vi "Lab Panel V5.11.vi"() -> ()   [LabVIEW 2013] (continued)
                      }
                    }
                    n1129 = Increment(x=w2164) -> (x+1=w2165:dbl)
                    n1130 = Greater Or Equal?(x=w2172, y=w2165) -> (x >= y?=w2174:bool)
                    n1131 = case shown="True" w2174 {
                      tunnel: w2169 -> [w2184 _]
                      tunnel: w2168 -> [w2183 _]
                      tunnel: w2167 -> [w2182 _]
                      tunnel: w2166 -> [w2181 _]
                      frame True {
                        n1132 = stacked-sequence {
                          tunnel: w2184 -> [w2188 _]
                          tunnel: w2183 -> [w2186 w2192]
                          tunnel: w2182 -> [_ w2195]
                          tunnel: w2181 -> [w2185 _]
                          frame #0 {
                            n1133 = Build Array(w2186) -> (w2189:string[])
                            n1134 = Build Array(w2188) -> (w2187:dbl[])
                            n1135 = TDMS Write(0:w2185, 5:"TEST PASS", 7:w2189, 9:w2187) -> (15:w2191:errorcluster)  [unwired: 2 in, 3 out]
                            n1136 = local write "data file error"(w2191) -> ()
                          }
                          frame #1 {
                            n1137 = Bundle(cluster=w2195, "STATUS"=w2192) -> (w2193:T4)  [unwired: 2 in]
                            n1138 = local write "RESULT LAB02-1"(TRUE) -> ()
                            n1139 = local write "DISP LAB02-1"(w2193) -> ()
                          }
                        }
                      }
                      frame False {
                      }
                    }
                  }
                }
              }
              frame #3 {
                # "LAB02-2"
                n1140 = Less?(x=w2196, y=2) -> (x < y?=w2199:bool)
                n1141 = local read "DISP LAB02-2"() -> (w2201:T4)
                n1142 = Unbundle(w2201) -> ("STATUS"=w2202:string)  [unwired: 2 out]
                n1143 = Equal?(x=w2202, y="RUN") -> (x = y?=w2198:bool)
                n1144 = And(x=w2198, y=w2199) -> (x .and. y?=w2197:bool)
                n1145 = case shown="True" w2197 {
                  tunnel: w2201 -> [_ w2207]
                  tunnel: w2196 -> [_ w2211]
                  frame False {
                  }
                  frame True {
                    n1146 = local read "SET LAB02-2"() -> (w2213:T5)
                    n1147 = local read "TDMS LAB02-2"() -> (w2206:refnum<k34>)
                    n1148 = Unbundle(w2207) -> ("CYCLE"=w2212:dbl)  [unwired: 2 out]
                    n1149 = Unbundle(w2213) -> ("CYCLES"=w2204:dbl, "T-RISE mins"=w2210:dbl)  [unwired: 3 out]
                    n1150 = case shown="\"T-RISE TEST\"" w2211 {
                      tunnel: w2210 -> [_ _ w2220]
                      tunnel: [w2215 w2217 w2220] -> w2209
                      tunnel: w2204 -> [w2215 w2217 _]
                      tunnel: ["CHART PASS" "CYCLE PASS" "T-RISE PASS"] -> w2208
                      frame "CHART TEST", Default {
                      }
                      frame "CYCLE TEST" {
                      }
                      frame "T-RISE TEST" {
                      }
                    }
                    n1151 = Increment(x=w2204) -> (x+1=w2205:dbl)
                    n1152 = Greater Or Equal?(x=w2212, y=w2205) -> (x >= y?=w2214:bool)
                    n1153 = case shown="True" w2214 {
                      tunnel: w2209 -> [w2224 _]
                      tunnel: w2208 -> [w2223 _]
                      tunnel: w2207 -> [w2222 _]
                      tunnel: w2206 -> [w2221 _]
                      frame True {
                        n1154 = stacked-sequence {
                          tunnel: w2224 -> [w2228 _]
                          tunnel: w2223 -> [w2226 w2232]
                          tunnel: w2222 -> [_ w2235]
                          tunnel: w2221 -> [w2225 _]
                          frame #0 {
                            n1155 = Build Array(w2226) -> (w2229:string[])
                            n1156 = Build Array(w2228) -> (w2227:dbl[])
                            n1157 = TDMS Write(0:w2225, 5:"TEST PASS", 7:w2229, 9:w2227) -> (15:w2231:errorcluster)  [unwired: 2 in, 3 out]
                            n1158 = local write "data file error"(w2231) -> ()
                          }
                          frame #1 {
                            n1159 = Bundle(cluster=w2235, "STATUS"=w2232) -> (w2233:T4)  [unwired: 2 in]
                            n1160 = local write "RESULT LAB02-2"(TRUE) -> ()
                            n1161 = local write "DISP LAB02-2"(w2233) -> ()
                          }
                        }
                      }
                      frame False {
                      }
                    }
                  }
                }
              }
              frame #4 {
                # "LAB03-1"
                n1162 = Less?(x=w2236, y=2) -> (x < y?=w2239:bool)
                n1163 = local read "DISP LAB03-1"() -> (w2241:T4)
                n1164 = Unbundle(w2241) -> ("STATUS"=w2242:string)  [unwired: 2 out]
                n1165 = Equal?(x=w2242, y="RUN") -> (x = y?=w2238:bool)
                n1166 = And(x=w2238, y=w2239) -> (x .and. y?=w2237:bool)
                n1167 = case shown="True" w2237 {
                  tunnel: w2241 -> [_ w2247]
                  tunnel: w2236 -> [_ w2251]
                  frame False {
                  }
                  frame True {
                    n1168 = local read "SET LAB03-1"() -> (w2253:T5)
                    n1169 = local read "TDMS LAB03-1"() -> (w2246:refnum<k34>)
                    n1170 = Unbundle(w2247) -> ("CYCLE"=w2252:dbl)  [unwired: 2 out]
                    n1171 = Unbundle(w2253) -> ("CYCLES"=w2244:dbl, "T-RISE mins"=w2250:dbl)  [unwired: 3 out]
                    n1172 = case shown="\"T-RISE TEST\"" w2251 {
                      tunnel: w2250 -> [_ _ w2260]
                      tunnel: [w2255 w2257 w2260] -> w2249
                      tunnel: w2244 -> [w2255 w2257 _]
                      tunnel: ["CHART PASS" "CYCLE PASS" "T-RISE PASS"] -> w2248
                      frame "CHART TEST", Default {
                      }
                      frame "CYCLE TEST" {
                      }
                      frame "T-RISE TEST" {
                      }
                    }
                    n1173 = Increment(x=w2244) -> (x+1=w2245:dbl)
                    n1174 = Greater Or Equal?(x=w2252, y=w2245) -> (x >= y?=w2254:bool)
                    n1175 = case shown="True" w2254 {
                      tunnel: w2249 -> [w2264 _]
                      tunnel: w2248 -> [w2263 _]
                      tunnel: w2247 -> [w2262 _]
                      tunnel: w2246 -> [w2261 _]
                      frame True {
                        n1176 = stacked-sequence {
                          tunnel: w2264 -> [w2268 _]
                          tunnel: w2263 -> [w2266 w2272]
                          tunnel: w2262 -> [_ w2275]
                          tunnel: w2261 -> [w2265 _]
                          frame #0 {
                            n1177 = Build Array(w2266) -> (w2269:string[])
                            n1178 = Build Array(w2268) -> (w2267:dbl[])
                            n1179 = TDMS Write(0:w2265, 5:"TEST PASS", 7:w2269, 9:w2267) -> (15:w2271:errorcluster)  [unwired: 2 in, 3 out]
                            n1180 = local write "data file error"(w2271) -> ()
                          }
                          frame #1 {
                            n1181 = Bundle(cluster=w2275, "STATUS"=w2272) -> (w2273:T4)  [unwired: 2 in]
                            n1182 = local write "RESULT LAB03-1"(TRUE) -> ()
                            n1183 = local write "DISP LAB03-1"(w2273) -> ()
                          }
                        }
                      }
                      frame False {
                      }
                    }
                  }
                }
              }
              frame #5 {
                # "LAB03-2"
                n1184 = Less?(x=w2276, y=2) -> (x < y?=w2279:bool)
                n1185 = local read "DISP LAB03-2"() -> (w2281:T4)
                n1186 = Unbundle(w2281) -> ("STATUS"=w2282:string)  [unwired: 2 out]
                n1187 = Equal?(x=w2282, y="RUN") -> (x = y?=w2278:bool)
                n1188 = And(x=w2278, y=w2279) -> (x .and. y?=w2277:bool)
                n1189 = case shown="True" w2277 {
                  tunnel: w2281 -> [_ w2287]
                  tunnel: w2276 -> [_ w2291]
                  frame False {
                  }
                  frame True {
                    n1190 = local read "SET LAB03-2"() -> (w2293:T5)
                    n1191 = local read "TDMS LAB03-2"() -> (w2286:refnum<k34>)
                    n1192 = Unbundle(w2287) -> ("CYCLE"=w2292:dbl)  [unwired: 2 out]
                    n1193 = Unbundle(w2293) -> ("CYCLES"=w2284:dbl, "T-RISE mins"=w2290:dbl)  [unwired: 3 out]
                    n1194 = case shown="\"T-RISE TEST\"" w2291 {
                      tunnel: w2290 -> [_ _ w2300]
                      tunnel: [w2295 w2297 w2300] -> w2289
                      tunnel: w2284 -> [w2295 w2297 _]
                      tunnel: ["CHART PASS" "CYCLE PASS" "T-RISE PASS"] -> w2288
                      frame "CHART TEST", Default {
                      }
                      frame "CYCLE TEST" {
                      }
                      frame "T-RISE TEST" {
                      }
                    }
                    n1195 = Increment(x=w2284) -> (x+1=w2285:dbl)
                    n1196 = Greater Or Equal?(x=w2292, y=w2285) -> (x >= y?=w2294:bool)
                    n1197 = case shown="True" w2294 {
                      tunnel: w2289 -> [w2304 _]
                      tunnel: w2288 -> [w2303 _]
                      tunnel: w2287 -> [w2302 _]
                      tunnel: w2286 -> [w2301 _]
                      frame True {
                        n1198 = stacked-sequence {
                          tunnel: w2304 -> [w2308 _]
                          tunnel: w2303 -> [w2306 w2312]
                          tunnel: w2302 -> [_ w2315]
                          tunnel: w2301 -> [w2305 _]
                          frame #0 {
                            n1199 = Build Array(w2306) -> (w2309:string[])
                            n1200 = Build Array(w2308) -> (w2307:dbl[])
                            n1201 = TDMS Write(0:w2305, 5:"TEST PASS", 7:w2309, 9:w2307) -> (15:w2311:errorcluster)  [unwired: 2 in, 3 out]
                            n1202 = local write "data file error"(w2311) -> ()
                          }
                          frame #1 {
                            n1203 = Bundle(cluster=w2315, "STATUS"=w2312) -> (w2313:T4)  [unwired: 2 in]
                            n1204 = local write "RESULT LAB03-2"(TRUE) -> ()
                            n1205 = local write "DISP LAB03-2"(w2313) -> ()
                          }
                        }
                      }
                      frame False {
                      }
                    }
                  }
                }
              }
              frame #6 {
                # "LAB04-1"
                n1206 = Less?(x=w2316, y=2) -> (x < y?=w2319:bool)
                n1207 = local read "DISP LAB04-1"() -> (w2321:T4)
                n1208 = Unbundle(w2321) -> ("STATUS"=w2322:string)  [unwired: 2 out]
                n1209 = Equal?(x=w2322, y="RUN") -> (x = y?=w2318:bool)
                n1210 = And(x=w2318, y=w2319) -> (x .and. y?=w2317:bool)
                n1211 = case shown="True" w2317 {
                  tunnel: w2321 -> [_ w2327]
                  tunnel: w2316 -> [_ w2331]
                  frame False {
                  }
                  frame True {
                    n1212 = local read "SET LAB04-1"() -> (w2333:T5)
                    n1213 = local read "TDMS LAB04-1"() -> (w2326:refnum<k34>)
                    n1214 = Unbundle(w2327) -> ("CYCLE"=w2332:dbl)  [unwired: 2 out]
                    n1215 = Unbundle(w2333) -> ("CYCLES"=w2324:dbl, "T-RISE mins"=w2330:dbl)  [unwired: 3 out]
                    n1216 = case shown="\"T-RISE TEST\"" w2331 {
                      tunnel: w2330 -> [_ _ w2340]
                      tunnel: [w2335 w2337 w2340] -> w2329
                      tunnel: w2324 -> [w2335 w2337 _]
                      tunnel: ["CHART PASS" "CYCLE PASS" "T-RISE PASS"] -> w2328
                      frame "CHART TEST", Default {
                      }
                      frame "CYCLE TEST" {
                      }
                      frame "T-RISE TEST" {
                      }
                    }
                    n1217 = Increment(x=w2324) -> (x+1=w2325:dbl)
                    n1218 = Greater Or Equal?(x=w2332, y=w2325) -> (x >= y?=w2334:bool)
                    n1219 = case shown="True" w2334 {
                      tunnel: w2329 -> [w2344 _]
                      tunnel: w2328 -> [w2343 _]
                      tunnel: w2327 -> [w2342 _]
                      tunnel: w2326 -> [w2341 _]
                      frame True {
                        n1220 = stacked-sequence {
                          tunnel: w2344 -> [w2348 _]
                          tunnel: w2343 -> [w2346 w2352]
                          tunnel: w2342 -> [_ w2355]
                          tunnel: w2341 -> [w2345 _]
                          frame #0 {
                            n1221 = Build Array(w2346) -> (w2349:string[])
                            n1222 = Build Array(w2348) -> (w2347:dbl[])
                            n1223 = TDMS Write(0:w2345, 5:"TEST PASS", 7:w2349, 9:w2347) -> (15:w2351:errorcluster)  [unwired: 2 in, 3 out]
                            n1224 = local write "data file error"(w2351) -> ()
                          }
                          frame #1 {
                            n1225 = Bundle(cluster=w2355, "STATUS"=w2352) -> (w2353:T4)  [unwired: 2 in]
                            n1226 = local write "RESULT LAB04-1"(TRUE) -> ()
                            n1227 = local write "DISP LAB04-1"(w2353) -> ()
                          }
                        }
                      }
                      frame False {
                      }
                    }
                  }
                }
              }
              frame #7 {
                # "LAB04-2"
                n1228 = Less?(x=w2356, y=2) -> (x < y?=w2359:bool)
                n1229 = local read "DISP LAB04-2"() -> (w2361:T4)
                n1230 = Unbundle(w2361) -> ("STATUS"=w2362:string)  [unwired: 2 out]
                n1231 = Equal?(x=w2362, y="RUN") -> (x = y?=w2358:bool)
                n1232 = And(x=w2358, y=w2359) -> (x .and. y?=w2357:bool)
                n1233 = case shown="True" w2357 {
                  tunnel: w2361 -> [_ w2367]
                  tunnel: w2356 -> [_ w2371]
                  frame False {
                  }
                  frame True {
                    n1234 = local read "SET LAB04-2"() -> (w2373:T5)
                    n1235 = local read "TDMS LAB04-2"() -> (w2366:refnum<k34>)
                    n1236 = Unbundle(w2367) -> ("CYCLE"=w2372:dbl)  [unwired: 2 out]
                    n1237 = Unbundle(w2373) -> ("CYCLES"=w2364:dbl, "T-RISE mins"=w2370:dbl)  [unwired: 3 out]
                    n1238 = case shown="\"T-RISE TEST\"" w2371 {
                      tunnel: w2370 -> [_ _ w2380]
                      tunnel: [w2375 w2377 w2380] -> w2369
                      tunnel: w2364 -> [w2375 w2377 _]
                      tunnel: ["CHART PASS" "CYCLE PASS" "T-RISE PASS"] -> w2368
                      frame "CHART TEST", Default {
                      }
                      frame "CYCLE TEST" {
                      }
                      frame "T-RISE TEST" {
                      }
                    }
                    n1239 = Increment(x=w2364) -> (x+1=w2365:dbl)
                    n1240 = Greater Or Equal?(x=w2372, y=w2365) -> (x >= y?=w2374:bool)
                    n1241 = case shown="True" w2374 {
                      tunnel: w2369 -> [w2384 _]
                      tunnel: w2368 -> [w2383 _]
                      tunnel: w2367 -> [w2382 _]
                      tunnel: w2366 -> [w2381 _]
                      frame True {
                        n1242 = stacked-sequence {
                          tunnel: w2384 -> [w2388 _]
                          tunnel: w2383 -> [w2386 w2392]
                          tunnel: w2382 -> [_ w2395]
                          tunnel: w2381 -> [w2385 _]
                          frame #0 {
                            n1243 = Build Array(w2386) -> (w2389:string[])
                            n1244 = Build Array(w2388) -> (w2387:dbl[])
                            n1245 = TDMS Write(0:w2385, 5:"TEST PASS", 7:w2389, 9:w2387) -> (15:w2391:errorcluster)  [unwired: 2 in, 3 out]
                            n1246 = local write "data file error"(w2391) -> ()
                          }
                          frame #1 {
                            n1247 = Bundle(cluster=w2395, "STATUS"=w2392) -> (w2393:T4)  [unwired: 2 in]
                            n1248 = local write "RESULT LAB04-2"(TRUE) -> ()
                            n1249 = local write "DISP LAB04-2"(w2393) -> ()
                          }
                        }
                      }
                      frame False {
                      }
                    }
                  }
                }
              }
              frame #8 {
                # "LAB05-1"
                n1250 = Less?(x=w2396, y=2) -> (x < y?=w2399:bool)
                n1251 = local read "DISP LAB05-1"() -> (w2401:T4)
                n1252 = Unbundle(w2401) -> ("STATUS"=w2402:string)  [unwired: 2 out]
                n1253 = Equal?(x=w2402, y="RUN") -> (x = y?=w2398:bool)
                n1254 = And(x=w2398, y=w2399) -> (x .and. y?=w2397:bool)
                n1255 = case shown="True" w2397 {
                  tunnel: w2401 -> [_ w2407]
                  tunnel: w2396 -> [_ w2411]
                  frame False {
                  }
                  frame True {
                    n1256 = local read "SET LAB05-1"() -> (w2413:T5)
                    n1257 = local read "TDMS LAB05-1"() -> (w2406:refnum<k34>)
                    n1258 = Unbundle(w2407) -> ("CYCLE"=w2412:dbl)  [unwired: 2 out]
                    n1259 = Unbundle(w2413) -> ("CYCLES"=w2404:dbl, "T-RISE mins"=w2410:dbl)  [unwired: 3 out]
                    n1260 = case shown="\"T-RISE TEST\"" w2411 {
                      tunnel: w2410 -> [_ _ w2420]
                      tunnel: [w2415 w2417 w2420] -> w2409
                      tunnel: w2404 -> [w2415 w2417 _]
                      tunnel: ["CHART PASS" "CYCLE PASS" "T-RISE PASS"] -> w2408
                      frame "CHART TEST", Default {
                      }
                      frame "CYCLE TEST" {
                      }
                      frame "T-RISE TEST" {
                      }
                    }
                    n1261 = Increment(x=w2404) -> (x+1=w2405:dbl)
                    n1262 = Greater Or Equal?(x=w2412, y=w2405) -> (x >= y?=w2414:bool)
                    n1263 = case shown="True" w2414 {
                      tunnel: w2409 -> [w2424 _]
                      tunnel: w2408 -> [w2423 _]
                      tunnel: w2407 -> [w2422 _]
                      tunnel: w2406 -> [w2421 _]
                      frame True {
                        n1264 = stacked-sequence {
                          tunnel: w2424 -> [w2428 _]
                          tunnel: w2423 -> [w2426 w2432]
                          tunnel: w2422 -> [_ w2435]
                          tunnel: w2421 -> [w2425 _]
                          frame #0 {
                            n1265 = Build Array(w2426) -> (w2429:string[])
                            n1266 = Build Array(w2428) -> (w2427:dbl[])
                            n1267 = TDMS Write(0:w2425, 5:"TEST PASS", 7:w2429, 9:w2427) -> (15:w2431:errorcluster)  [unwired: 2 in, 3 out]
                            n1268 = local write "data file error"(w2431) -> ()
                          }
                          frame #1 {
                            n1269 = Bundle(cluster=w2435, "STATUS"=w2432) -> (w2433:T4)  [unwired: 2 in]
                            n1270 = local write "RESULT LAB05-1"(TRUE) -> ()
                            n1271 = local write "DISP LAB05-1"(w2433) -> ()
                          }
                        }
                      }
                      frame False {
                      }
                    }
                  }
                }
              }
              frame #9 {
                # "LAB05-2"
                n1272 = Less?(x=w2436, y=2) -> (x < y?=w2439:bool)
                n1273 = local read "DISP LAB05-2"() -> (w2441:T4)
                n1274 = Unbundle(w2441) -> ("STATUS"=w2442:string)  [unwired: 2 out]
                n1275 = Equal?(x=w2442, y="RUN") -> (x = y?=w2438:bool)
                n1276 = And(x=w2438, y=w2439) -> (x .and. y?=w2437:bool)
                n1277 = case shown="True" w2437 {
                  tunnel: w2441 -> [_ w2447]
                  tunnel: w2436 -> [_ w2451]
                  frame False {
                  }
                  frame True {
                    n1278 = local read "SET LAB05-2"() -> (w2453:T5)
                    n1279 = local read "TDMS LAB05-2"() -> (w2446:refnum<k34>)
                    n1280 = Unbundle(w2447) -> ("CYCLE"=w2452:dbl)  [unwired: 2 out]
                    n1281 = Unbundle(w2453) -> ("CYCLES"=w2444:dbl, "T-RISE mins"=w2450:dbl)  [unwired: 3 out]
                    n1282 = case shown="\"T-RISE TEST\"" w2451 {
                      tunnel: w2450 -> [_ _ w2460]
                      tunnel: [w2455 w2457 w2460] -> w2449
                      tunnel: w2444 -> [w2455 w2457 _]
                      tunnel: ["CHART PASS" "CYCLE PASS" "T-RISE PASS"] -> w2448
                      frame "CHART TEST", Default {
                      }
                      frame "CYCLE TEST" {
                      }
                      frame "T-RISE TEST" {
                      }
                    }
                    n1283 = Increment(x=w2444) -> (x+1=w2445:dbl)
                    n1284 = Greater Or Equal?(x=w2452, y=w2445) -> (x >= y?=w2454:bool)
                    n1285 = case shown="True" w2454 {
                      tunnel: w2449 -> [w2464 _]
                      tunnel: w2448 -> [w2463 _]
                      tunnel: w2447 -> [w2462 _]
                      tunnel: w2446 -> [w2461 _]
                      frame True {
                        n1286 = stacked-sequence {
                          tunnel: w2464 -> [w2468 _]
                          tunnel: w2463 -> [w2466 w2472]
                          tunnel: w2462 -> [_ w2475]
                          tunnel: w2461 -> [w2465 _]
                          frame #0 {
                            n1287 = Build Array(w2466) -> (w2469:string[])
                            n1288 = Build Array(w2468) -> (w2467:dbl[])
                            n1289 = TDMS Write(0:w2465, 5:"TEST PASS", 7:w2469, 9:w2467) -> (15:w2471:errorcluster)  [unwired: 2 in, 3 out]
                            n1290 = local write "data file error"(w2471) -> ()
                          }
                          frame #1 {
                            n1291 = Bundle(cluster=w2475, "STATUS"=w2472) -> (w2473:T4)  [unwired: 2 in]
                            n1292 = local write "RESULT LAB05-2"(TRUE) -> ()
                            n1293 = local write "DISP LAB05-2"(w2473) -> ()
                          }
                        }
                      }
                      frame False {
                      }
                    }
                  }
                }
              }
            }
          }
          frame #5 {
            # "check if test cycles reached for temperature rise test"
            n1294 = stacked-sequence {
              tunnel: w2505 -> [_ _ _ _ _ _ _ _ _ _]
              tunnel: w2504 -> [_ _ _ _ _ _ _ _ _ _]
              tunnel: w2503 -> [_ _ _ _ _ _ _ _ _ _]
              tunnel: w2502 -> [_ _ _ _ _ _ _ _ _ _]
              tunnel: w2501 -> [_ _ _ _ _ _ _ _ _ _]
              tunnel: w2500 -> [_ _ _ _ _ _ _ _ _ _]
              tunnel: w2499 -> [_ _ _ _ _ _ _ _ _ _]
              tunnel: w2498 -> [_ _ _ _ _ _ _ _ _ _]
              tunnel: w2497 -> [_ _ _ _ _ _ _ _ _ _]
              tunnel: w2496 -> [_ _ _ _ _ _ _ _ _ _]
              tunnel: w2495 -> [w2511 _ _ _ _ _ _ _ _ _]
              tunnel: w2485 -> [w2506 _ _ _ _ _ _ _ _ _]
              tunnel: w2494 -> [_ w2537 _ _ _ _ _ _ _ _]
              tunnel: w2493 -> [_ _ w2567 _ _ _ _ _ _ _]
              tunnel: w2492 -> [_ _ _ w2597 _ _ _ _ _ _]
              tunnel: w2491 -> [_ _ _ _ w2627 _ _ _ _ _]
              tunnel: w2490 -> [_ _ _ _ _ w2657 _ _ _ _]
              tunnel: w2489 -> [_ _ _ _ _ _ w2687 _ _ _]
              tunnel: w2488 -> [_ _ _ _ _ _ _ w2717 _ _]
              tunnel: w2487 -> [_ _ _ _ _ _ _ _ w2747 _]
              tunnel: w2486 -> [_ _ _ _ _ _ _ _ _ w2777]
              tunnel: w2484 -> [_ w2536 _ _ _ _ _ _ _ _]
              tunnel: w2483 -> [_ _ w2566 _ _ _ _ _ _ _]
              tunnel: w2482 -> [_ _ _ w2596 _ _ _ _ _ _]
              tunnel: w2481 -> [_ _ _ _ w2626 _ _ _ _ _]
              tunnel: w2480 -> [_ _ _ _ _ w2656 _ _ _ _]
              tunnel: w2479 -> [_ _ _ _ _ _ w2686 _ _ _]
              tunnel: w2478 -> [_ _ _ _ _ _ _ w2716 _ _]
              tunnel: w2477 -> [_ _ _ _ _ _ _ _ w2746 _]
              tunnel: w2476 -> [_ _ _ _ _ _ _ _ _ w2776]
              frame #0 {
                # "LAB01-1"
                n1295 = Equal?(x=w2511, y=2) -> (x = y?=w2509:bool)
                n1296 = local read "DISP LAB01-1"() -> (w2512:T4)
                n1297 = Unbundle(w2512) -> ("STATUS"=w2513:string)  [unwired: 2 out]
                n1298 = Equal?(x=w2513, y="RUN") -> (x = y?=w2508:bool)
                n1299 = And(x=w2508, y=w2509) -> (x .and. y?=w2507:bool)
                n1300 = case shown="True" w2507 {
                  tunnel: w2512 -> [_ w2516]
                  tunnel: w2506 -> [_ w2519]
                  frame False {
                  }
                  frame True {
                    n1301 = local read "SET LAB01-1"() -> (w2518:T5)
                    n1302 = local read "TDMS LAB01-1"() -> (w2515:refnum<k34>)
                    n1303 = Unbundle(w2516) -> ("CYCLE"=w2520:dbl)  [unwired: 2 out]
                    n1304 = Unbundle(w2518) -> ("T-RISE mins"=w2517:dbl)  [unwired: 4 out]
                    n1305 = Greater Or Equal?(x=w2520, y=w2519) -> (x >= y?=w2521:bool)
                    n1306 = case shown="True" w2521 {
                      tunnel: w2517 -> [w2524 _]
                      tunnel: w2516 -> [w2523 _]
                      tunnel: w2515 -> [w2522 _]
                      frame True {
                        n1307 = stacked-sequence {
                          tunnel: w2524 -> [w2527 _]
                          tunnel: w2523 -> [_ w2532]
                          tunnel: w2522 -> [w2525 _]
                          frame #0 {
                            n1308 = Build Array("T-RISE") -> (w2529:string[])
                            n1309 = Build Array(w2527) -> (w2528:dbl[])
                            n1310 = TDMS Write(0:w2525, 5:"TEST PASS", 7:w2529, 9:w2528) -> (15:w2531:errorcluster)  [unwired: 2 in, 3 out]
                            n1311 = local write "data file error"(w2531) -> ()
                          }
                          frame #1 {
                            n1312 = Bundle(cluster=w2532, "STATUS"="T-RISE PASS") -> (w2534:T4)  [unwired: 2 in]
                            n1313 = local write "RESULT LAB01-1"(TRUE) -> ()
                            n1314 = local write "DISP LAB01-1"(w2534) -> ()
                          }
                        }
                      }
                      frame False {
                      }
                    }
                  }
                }
              }
              frame #1 {
                # "LAB01-2"
                n1315 = Equal?(x=w2537, y=2) -> (x = y?=w2540:bool)
                n1316 = local read "DISP LAB01-2"() -> (w2542:T4)
                n1317 = Unbundle(w2542) -> ("STATUS"=w2543:string)  [unwired: 2 out]
                n1318 = Equal?(x=w2543, y="RUN") -> (x = y?=w2539:bool)
                n1319 = And(x=w2539, y=w2540) -> (x .and. y?=w2538:bool)
                n1320 = case shown="True" w2538 {
                  tunnel: w2542 -> [_ w2546]
                  tunnel: w2536 -> [_ w2549]
                  frame False {
                  }
                  frame True {
                    n1321 = local read "SET LAB01-2"() -> (w2548:T5)
                    n1322 = local read "TDMS LAB01-2"() -> (w2545:refnum<k34>)
                    n1323 = Unbundle(w2546) -> ("CYCLE"=w2550:dbl)  [unwired: 2 out]
                    n1324 = Unbundle(w2548) -> ("T-RISE mins"=w2547:dbl)  [unwired: 4 out]
                    n1325 = Greater Or Equal?(x=w2550, y=w2549) -> (x >= y?=w2551:bool)
                    n1326 = case shown="True" w2551 {
                      tunnel: w2547 -> [w2554 _]
                      tunnel: w2546 -> [w2553 _]
                      tunnel: w2545 -> [w2552 _]
                      frame True {
                        n1327 = stacked-sequence {
                          tunnel: w2554 -> [w2557 _]
                          tunnel: w2553 -> [_ w2562]
                          tunnel: w2552 -> [w2555 _]
                          frame #0 {
                            n1328 = Build Array("T-RISE") -> (w2559:string[])
                            n1329 = Build Array(w2557) -> (w2558:dbl[])
                            n1330 = TDMS Write(0:w2555, 5:"TEST PASS", 7:w2559, 9:w2558) -> (15:w2561:errorcluster)  [unwired: 2 in, 3 out]
                            n1331 = local write "data file error"(w2561) -> ()
                          }
                          frame #1 {
                            n1332 = Bundle(cluster=w2562, "STATUS"="T-RISE PASS") -> (w2564:T4)  [unwired: 2 in]
                            n1333 = local write "RESULT LAB01-2"(TRUE) -> ()
                            n1334 = local write "DISP LAB01-2"(w2564) -> ()
                          }
                        }
                      }
                      frame False {
                      }
                    }
                  }
                }
              }
              frame #2 {
                # "LAB02-1"
                n1335 = Equal?(x=w2567, y=2) -> (x = y?=w2570:bool)
                n1336 = local read "DISP LAB02-1"() -> (w2572:T4)
                n1337 = Unbundle(w2572) -> ("STATUS"=w2573:string)  [unwired: 2 out]
                n1338 = Equal?(x=w2573, y="RUN") -> (x = y?=w2569:bool)
                n1339 = And(x=w2569, y=w2570) -> (x .and. y?=w2568:bool)
                n1340 = case shown="True" w2568 {
                  tunnel: w2572 -> [_ w2576]
                  tunnel: w2566 -> [_ w2579]
                  frame False {
                  }
                  frame True {
                    n1341 = local read "SET LAB02-1"() -> (w2578:T5)
                    n1342 = local read "TDMS LAB02-1"() -> (w2575:refnum<k34>)
                    n1343 = Unbundle(w2576) -> ("CYCLE"=w2580:dbl)  [unwired: 2 out]
                    n1344 = Unbundle(w2578) -> ("T-RISE mins"=w2577:dbl)  [unwired: 4 out]
                    n1345 = Greater Or Equal?(x=w2580, y=w2579) -> (x >= y?=w2581:bool)
                    n1346 = case shown="True" w2581 {
                      tunnel: w2577 -> [w2584 _]
                      tunnel: w2576 -> [w2583 _]
                      tunnel: w2575 -> [w2582 _]
                      frame True {
                        n1347 = stacked-sequence {
                          tunnel: w2584 -> [w2587 _]
                          tunnel: w2583 -> [_ w2592]
                          tunnel: w2582 -> [w2585 _]
                          frame #0 {
                            n1348 = Build Array("T-RISE") -> (w2589:string[])
                            n1349 = Build Array(w2587) -> (w2588:dbl[])
                            n1350 = TDMS Write(0:w2585, 5:"TEST PASS", 7:w2589, 9:w2588) -> (15:w2591:errorcluster)  [unwired: 2 in, 3 out]
                            n1351 = local write "data file error"(w2591) -> ()
                          }
                          frame #1 {
                            n1352 = Bundle(cluster=w2592, "STATUS"="T-RISE PASS") -> (w2594:T4)  [unwired: 2 in]
                            n1353 = local write "RESULT LAB02-1"(TRUE) -> ()
                            n1354 = local write "DISP LAB02-1"(w2594) -> ()
                          }
                        }
                      }
                      frame False {
                      }
                    }
                  }
                }
              }
              frame #3 {
                # "LAB02-2"
                n1355 = Equal?(x=w2597, y=2) -> (x = y?=w2600:bool)
                n1356 = local read "DISP LAB02-2"() -> (w2602:T4)
                n1357 = Unbundle(w2602) -> ("STATUS"=w2603:string)  [unwired: 2 out]
                n1358 = Equal?(x=w2603, y="RUN") -> (x = y?=w2599:bool)
                n1359 = And(x=w2599, y=w2600) -> (x .and. y?=w2598:bool)
                n1360 = case shown="True" w2598 {
                  tunnel: w2602 -> [_ w2606]
                  tunnel: w2596 -> [_ w2609]
                  frame False {
                  }
                  frame True {
                    n1361 = local read "SET LAB02-2"() -> (w2608:T5)
                    n1362 = local read "TDMS LAB02-2"() -> (w2605:refnum<k34>)
                    n1363 = Unbundle(w2606) -> ("CYCLE"=w2610:dbl)  [unwired: 2 out]
                    n1364 = Unbundle(w2608) -> ("T-RISE mins"=w2607:dbl)  [unwired: 4 out]
                    n1365 = Greater Or Equal?(x=w2610, y=w2609) -> (x >= y?=w2611:bool)
                    n1366 = case shown="True" w2611 {
                      tunnel: w2607 -> [w2614 _]
                      tunnel: w2606 -> [w2613 _]
                      tunnel: w2605 -> [w2612 _]
                      frame True {
                        n1367 = stacked-sequence {
                          tunnel: w2614 -> [w2617 _]
                          tunnel: w2613 -> [_ w2622]
                          tunnel: w2612 -> [w2615 _]
                          frame #0 {
                            n1368 = Build Array("T-RISE") -> (w2619:string[])
                            n1369 = Build Array(w2617) -> (w2618:dbl[])
                            n1370 = TDMS Write(0:w2615, 5:"TEST PASS", 7:w2619, 9:w2618) -> (15:w2621:errorcluster)  [unwired: 2 in, 3 out]
                            n1371 = local write "data file error"(w2621) -> ()
                          }
                          frame #1 {
                            n1372 = Bundle(cluster=w2622, "STATUS"="T-RISE PASS") -> (w2624:T4)  [unwired: 2 in]
                            n1373 = local write "RESULT LAB02-2"(TRUE) -> ()
                            n1374 = local write "DISP LAB02-2"(w2624) -> ()
                          }
                        }
                      }
                      frame False {
                      }
                    }
                  }
                }
              }
              frame #4 {
                # "LAB03-1"
                n1375 = Equal?(x=w2627, y=2) -> (x = y?=w2630:bool)
                n1376 = local read "DISP LAB03-1"() -> (w2632:T4)
                n1377 = Unbundle(w2632) -> ("STATUS"=w2633:string)  [unwired: 2 out]
                n1378 = Equal?(x=w2633, y="RUN") -> (x = y?=w2629:bool)
                n1379 = And(x=w2629, y=w2630) -> (x .and. y?=w2628:bool)
                n1380 = case shown="True" w2628 {
                  tunnel: w2632 -> [_ w2636]
                  tunnel: w2626 -> [_ w2639]
                  frame False {
                  }
                  frame True {
                    n1381 = local read "SET LAB03-1"() -> (w2638:T5)
                    n1382 = local read "TDMS LAB03-1"() -> (w2635:refnum<k34>)
                    n1383 = Unbundle(w2636) -> ("CYCLE"=w2640:dbl)  [unwired: 2 out]
                    n1384 = Unbundle(w2638) -> ("T-RISE mins"=w2637:dbl)  [unwired: 4 out]
                    n1385 = Greater Or Equal?(x=w2640, y=w2639) -> (x >= y?=w2641:bool)
                    n1386 = case shown="True" w2641 {
                      tunnel: w2637 -> [w2644 _]
                      tunnel: w2636 -> [w2643 _]
                      tunnel: w2635 -> [w2642 _]
                      frame True {
                        n1387 = stacked-sequence {
                          tunnel: w2644 -> [w2647 _]
                          tunnel: w2643 -> [_ w2652]
                          tunnel: w2642 -> [w2645 _]
                          frame #0 {
                            n1388 = Build Array("T-RISE") -> (w2649:string[])
                            n1389 = Build Array(w2647) -> (w2648:dbl[])
                            n1390 = TDMS Write(0:w2645, 5:"TEST PASS", 7:w2649, 9:w2648) -> (15:w2651:errorcluster)  [unwired: 2 in, 3 out]
                            n1391 = local write "data file error"(w2651) -> ()
                          }
                          frame #1 {
                            n1392 = Bundle(cluster=w2652, "STATUS"="T-RISE PASS") -> (w2654:T4)  [unwired: 2 in]
                            n1393 = local write "RESULT LAB03-1"(TRUE) -> ()
                            n1394 = local write "DISP LAB03-1"(w2654) -> ()
                          }
                        }
                      }
                      frame False {
                      }
                    }
                  }
                }
              }
              frame #5 {
                # "LAB03-2"
                n1395 = Equal?(x=w2657, y=2) -> (x = y?=w2660:bool)
                n1396 = local read "DISP LAB03-2"() -> (w2662:T4)
                n1397 = Unbundle(w2662) -> ("STATUS"=w2663:string)  [unwired: 2 out]
                n1398 = Equal?(x=w2663, y="RUN") -> (x = y?=w2659:bool)
                n1399 = And(x=w2659, y=w2660) -> (x .and. y?=w2658:bool)
                n1400 = case shown="True" w2658 {
                  tunnel: w2662 -> [_ w2666]
                  tunnel: w2656 -> [_ w2669]
                  frame False {
                  }
                  frame True {
                    n1401 = local read "SET LAB03-2"() -> (w2668:T5)
                    n1402 = local read "TDMS LAB03-2"() -> (w2665:refnum<k34>)
                    n1403 = Unbundle(w2666) -> ("CYCLE"=w2670:dbl)  [unwired: 2 out]
                    n1404 = Unbundle(w2668) -> ("T-RISE mins"=w2667:dbl)  [unwired: 4 out]
                    n1405 = Greater Or Equal?(x=w2670, y=w2669) -> (x >= y?=w2671:bool)
                    n1406 = case shown="True" w2671 {
                      tunnel: w2667 -> [w2674 _]
                      tunnel: w2666 -> [w2673 _]
                      tunnel: w2665 -> [w2672 _]
                      frame True {
                        n1407 = stacked-sequence {
                          tunnel: w2674 -> [w2677 _]
                          tunnel: w2673 -> [_ w2682]
                          tunnel: w2672 -> [w2675 _]
                          frame #0 {
                            n1408 = Build Array("T-RISE") -> (w2679:string[])
                            n1409 = Build Array(w2677) -> (w2678:dbl[])
                            n1410 = TDMS Write(0:w2675, 5:"TEST PASS", 7:w2679, 9:w2678) -> (15:w2681:errorcluster)  [unwired: 2 in, 3 out]
                            n1411 = local write "data file error"(w2681) -> ()
                          }
                          frame #1 {
                            n1412 = Bundle(cluster=w2682, "STATUS"="T-RISE PASS") -> (w2684:T4)  [unwired: 2 in]
                            n1413 = local write "RESULT LAB03-2"(TRUE) -> ()
                            n1414 = local write "DISP LAB03-2"(w2684) -> ()
                          }
                        }
                      }
                      frame False {
                      }
                    }
                  }
                }
              }
              frame #6 {
                # "LAB04-1"
                n1415 = Equal?(x=w2687, y=2) -> (x = y?=w2690:bool)
                n1416 = local read "DISP LAB04-1"() -> (w2692:T4)
                n1417 = Unbundle(w2692) -> ("STATUS"=w2693:string)  [unwired: 2 out]
                n1418 = Equal?(x=w2693, y="RUN") -> (x = y?=w2689:bool)
                n1419 = And(x=w2689, y=w2690) -> (x .and. y?=w2688:bool)
                n1420 = case shown="True" w2688 {
                  tunnel: w2692 -> [_ w2696]
                  tunnel: w2686 -> [_ w2699]
                  frame False {
                  }
                  frame True {
                    n1421 = local read "SET LAB04-1"() -> (w2698:T5)
                    n1422 = local read "TDMS LAB04-1"() -> (w2695:refnum<k34>)
                    n1423 = Unbundle(w2696) -> ("CYCLE"=w2700:dbl)  [unwired: 2 out]
                    n1424 = Unbundle(w2698) -> ("T-RISE mins"=w2697:dbl)  [unwired: 4 out]
                    n1425 = Greater Or Equal?(x=w2700, y=w2699) -> (x >= y?=w2701:bool)
                    n1426 = case shown="True" w2701 {
                      tunnel: w2697 -> [w2704 _]
                      tunnel: w2696 -> [w2703 _]
                      tunnel: w2695 -> [w2702 _]
                      frame True {
                        n1427 = stacked-sequence {
                          tunnel: w2704 -> [w2707 _]
                          tunnel: w2703 -> [_ w2712]
                          tunnel: w2702 -> [w2705 _]
                          frame #0 {
                            n1428 = Build Array("T-RISE") -> (w2709:string[])
                            n1429 = Build Array(w2707) -> (w2708:dbl[])
                            n1430 = TDMS Write(0:w2705, 5:"TEST PASS", 7:w2709, 9:w2708) -> (15:w2711:errorcluster)  [unwired: 2 in, 3 out]
                            n1431 = local write "data file error"(w2711) -> ()
                          }
                          frame #1 {
                            n1432 = Bundle(cluster=w2712, "STATUS"="T-RISE PASS") -> (w2714:T4)  [unwired: 2 in]
                            n1433 = local write "RESULT LAB04-1"(TRUE) -> ()
                            n1434 = local write "DISP LAB04-1"(w2714) -> ()
                          }
                        }
                      }
                      frame False {
                      }
                    }
                  }
                }
              }
              frame #7 {
                # "LAB04-2"
                n1435 = Equal?(x=w2717, y=2) -> (x = y?=w2720:bool)
                n1436 = local read "DISP LAB04-2"() -> (w2722:T4)
                n1437 = Unbundle(w2722) -> ("STATUS"=w2723:string)  [unwired: 2 out]
                n1438 = Equal?(x=w2723, y="RUN") -> (x = y?=w2719:bool)
                n1439 = And(x=w2719, y=w2720) -> (x .and. y?=w2718:bool)
                n1440 = case shown="True" w2718 {
                  tunnel: w2722 -> [_ w2726]
                  tunnel: w2716 -> [_ w2729]
                  frame False {
                  }
                  frame True {
                    n1441 = local read "SET LAB04-2"() -> (w2728:T5)
                    n1442 = local read "TDMS LAB04-2"() -> (w2725:refnum<k34>)
                    n1443 = Unbundle(w2726) -> ("CYCLE"=w2730:dbl)  [unwired: 2 out]
                    n1444 = Unbundle(w2728) -> ("T-RISE mins"=w2727:dbl)  [unwired: 4 out]
                    n1445 = Greater Or Equal?(x=w2730, y=w2729) -> (x >= y?=w2731:bool)
                    n1446 = case shown="True" w2731 {
                      tunnel: w2727 -> [w2734 _]
                      tunnel: w2726 -> [w2733 _]
                      tunnel: w2725 -> [w2732 _]
                      frame True {
                        n1447 = stacked-sequence {
                          tunnel: w2734 -> [w2737 _]
                          tunnel: w2733 -> [_ w2742]
                          tunnel: w2732 -> [w2735 _]
                          frame #0 {
                            n1448 = Build Array("T-RISE") -> (w2739:string[])
                            n1449 = Build Array(w2737) -> (w2738:dbl[])
                            n1450 = TDMS Write(0:w2735, 5:"TEST PASS", 7:w2739, 9:w2738) -> (15:w2741:errorcluster)  [unwired: 2 in, 3 out]
                            n1451 = local write "data file error"(w2741) -> ()
                          }
                          frame #1 {
                            n1452 = Bundle(cluster=w2742, "STATUS"="T-RISE PASS") -> (w2744:T4)  [unwired: 2 in]
                            n1453 = local write "RESULT LAB04-2"(TRUE) -> ()
                            n1454 = local write "DISP LAB04-2"(w2744) -> ()
                          }
                        }
                      }
                      frame False {
                      }
                    }
                  }
                }
              }
              frame #8 {
                # "LAB05-1"
                n1455 = Equal?(x=w2747, y=2) -> (x = y?=w2750:bool)
                n1456 = local read "DISP LAB05-1"() -> (w2752:T4)
                n1457 = Unbundle(w2752) -> ("STATUS"=w2753:string)  [unwired: 2 out]
                n1458 = Equal?(x=w2753, y="RUN") -> (x = y?=w2749:bool)
                n1459 = And(x=w2749, y=w2750) -> (x .and. y?=w2748:bool)
                n1460 = case shown="True" w2748 {
                  tunnel: w2752 -> [_ w2756]
                  tunnel: w2746 -> [_ w2759]
                  frame False {
                  }
                  frame True {
                    n1461 = local read "SET LAB05-1"() -> (w2758:T5)
                    n1462 = local read "TDMS LAB05-1"() -> (w2755:refnum<k34>)
                    n1463 = Unbundle(w2756) -> ("CYCLE"=w2760:dbl)  [unwired: 2 out]
                    n1464 = Unbundle(w2758) -> ("T-RISE mins"=w2757:dbl)  [unwired: 4 out]
                    n1465 = Greater Or Equal?(x=w2760, y=w2759) -> (x >= y?=w2761:bool)
                    n1466 = case shown="True" w2761 {
                      tunnel: w2757 -> [w2764 _]
                      tunnel: w2756 -> [w2763 _]
                      tunnel: w2755 -> [w2762 _]
                      frame True {
                        n1467 = stacked-sequence {
                          tunnel: w2764 -> [w2767 _]
                          tunnel: w2763 -> [_ w2772]
                          tunnel: w2762 -> [w2765 _]
                          frame #0 {
                            n1468 = Build Array("T-RISE") -> (w2769:string[])
                            n1469 = Build Array(w2767) -> (w2768:dbl[])
                            n1470 = TDMS Write(0:w2765, 5:"TEST PASS", 7:w2769, 9:w2768) -> (15:w2771:errorcluster)  [unwired: 2 in, 3 out]
                            n1471 = local write "data file error"(w2771) -> ()
                          }
                          frame #1 {
                            n1472 = Bundle(cluster=w2772, "STATUS"="T-RISE PASS") -> (w2774:T4)  [unwired: 2 in]
                            n1473 = local write "RESULT LAB05-1"(TRUE) -> ()
                            n1474 = local write "DISP LAB05-1"(w2774) -> ()
                          }
                        }
                      }
                      frame False {
                      }
                    }
                  }
                }
              }
              frame #9 {
                # "LAB05-2"
                n1475 = Equal?(x=w2777, y=2) -> (x = y?=w2780:bool)
                n1476 = local read "DISP LAB05-2"() -> (w2782:T4)
                n1477 = Unbundle(w2782) -> ("STATUS"=w2783:string)  [unwired: 2 out]
                n1478 = Equal?(x=w2783, y="RUN") -> (x = y?=w2779:bool)
                n1479 = And(x=w2779, y=w2780) -> (x .and. y?=w2778:bool)
                n1480 = case shown="True" w2778 {
                  tunnel: w2782 -> [_ w2786]
                  tunnel: w2776 -> [_ w2789]
                  frame False {
                  }
                  frame True {
                    n1481 = local read "SET LAB05-2"() -> (w2788:T5)
                    n1482 = local read "TDMS LAB05-2"() -> (w2785:refnum<k34>)
                    n1483 = Unbundle(w2786) -> ("CYCLE"=w2790:dbl)  [unwired: 2 out]
                    n1484 = Unbundle(w2788) -> ("T-RISE mins"=w2787:dbl)  [unwired: 4 out]
                    n1485 = Greater Or Equal?(x=w2790, y=w2789) -> (x >= y?=w2791:bool)
                    n1486 = case shown="True" w2791 {
                      tunnel: w2787 -> [w2794 _]
                      tunnel: w2786 -> [w2793 _]
                      tunnel: w2785 -> [w2792 _]
                      frame True {
                        n1487 = stacked-sequence {
                          tunnel: w2794 -> [w2797 _]
                          tunnel: w2793 -> [_ w2802]
                          tunnel: w2792 -> [w2795 _]
                          frame #0 {
                            n1488 = Build Array("T-RISE") -> (w2799:string[])
                            n1489 = Build Array(w2797) -> (w2798:dbl[])
                            n1490 = TDMS Write(0:w2795, 5:"TEST PASS", 7:w2799, 9:w2798) -> (15:w2801:errorcluster)  [unwired: 2 in, 3 out]
                            n1491 = local write "data file error"(w2801) -> ()
                          }
                          frame #1 {
                            n1492 = Bundle(cluster=w2802, "STATUS"="T-RISE PASS") -> (w2804:T4)  [unwired: 2 in]
                            n1493 = local write "RESULT LAB05-2"(TRUE) -> ()
